vi "Trim Error Whitespace.vi"(1 "error in (no error)":errorcluster) -> (0 "error out":errorcluster)   [LabVIEW 2017, in "DSF Core.lvlib" / "Error Pointer.lvclass"]
uses:
  Pointers/Error/Error Pointer.lvclass
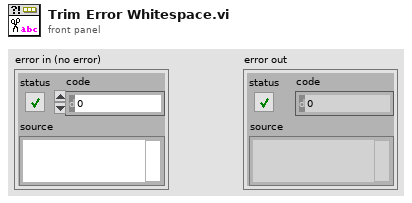
[diagram p1: front panel]
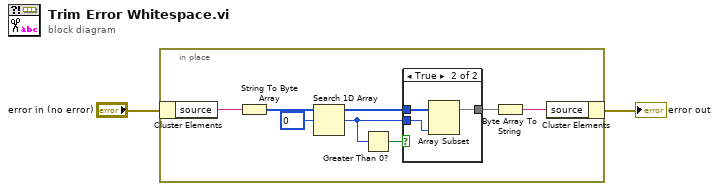
[diagram p0: block diagram]
diagram:
  n1 = in-place {
    n2 = in-place-cluster #1("error in (no error)") -> ("source"=w9:string)
    n3 = String To Byte Array(string=w9) -> (unsigned byte array=w5:u8[])
    n4 = Search 1D Array(1D array=w5, element=u8 0) -> (index of element=w4:i32)  [unwired: 1 in]
    n5 = Greater Than 0?(x=w4) -> (x > 0?=w3:bool)
    n6 = case shown="True" w3 {
      tunnel: [w10 w13] -> w7
      tunnel: w5 -> [w10 w12]
      tunnel: w4 -> [_ w11]
      frame False {
      }
      frame True {
        n7 = Array Subset(array=w12, length=w11) -> (w13:u8[])  [unwired: 1 in]
      }
    }
    n8 = Byte Array To String(unsigned byte array=w7) -> (string=w6:string)
    n9 = in-place-cluster #1("source"=w6) -> (→"error out":errorcluster)
  }
